vi "Read library name.vi"(8 "error in":errorcluster, 11 "editorscriptingobject in":refnum<class "editorscriptingobjectadvExService.lvclass">) -> (0 "error out":errorcluster, 2 "library name":string, 3 "editorscriptingobject out":refnum<class "editorscriptingobjectadvExService.lvclass">)   [LabVIEW 2013, in "editorscriptingobjectadvExService.lvclass"]
uses:
  editorscriptingobjectadvExService.lvclass
  editorscriptingobjectadvExService.lvclass/editorscriptingobjectadvExService.ctl
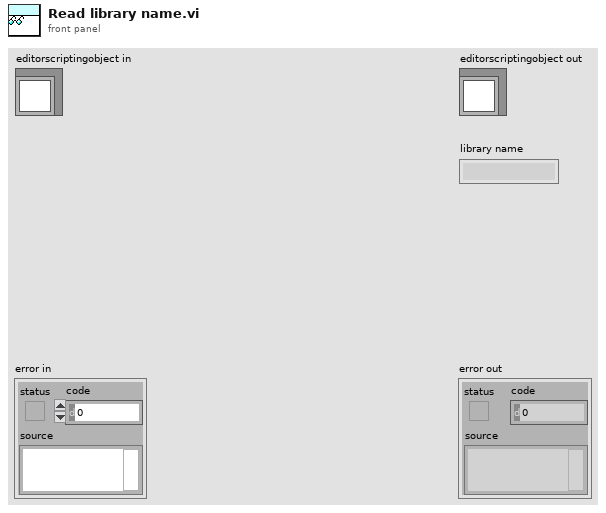
[diagram p1: front panel]
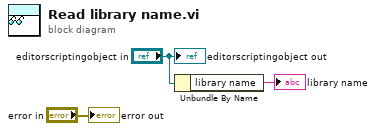
[diagram p0: block diagram]
diagram:
  n1 = Unbundle By Name("editorscriptingobject in") -> ("library name"=→"library name":string)
  "error out" <- "error in"
  "editorscriptingobject out" <- "editorscriptingobject in"
